vi "KPropertyTable Test.vi"() -> ()   [LabVIEW 2020]
uses:
  KPropertyTable/RowData.ctl
  KPropertyTable/DataType.ctl
  KPropertyTable/KPropertyTable.xctl
panel:
  out "data":T1
  in  "stop":bool
  in  "Table":T2[](xcontrol)
  out "Rows":T2[](array[typedef])
  in  "props":T1
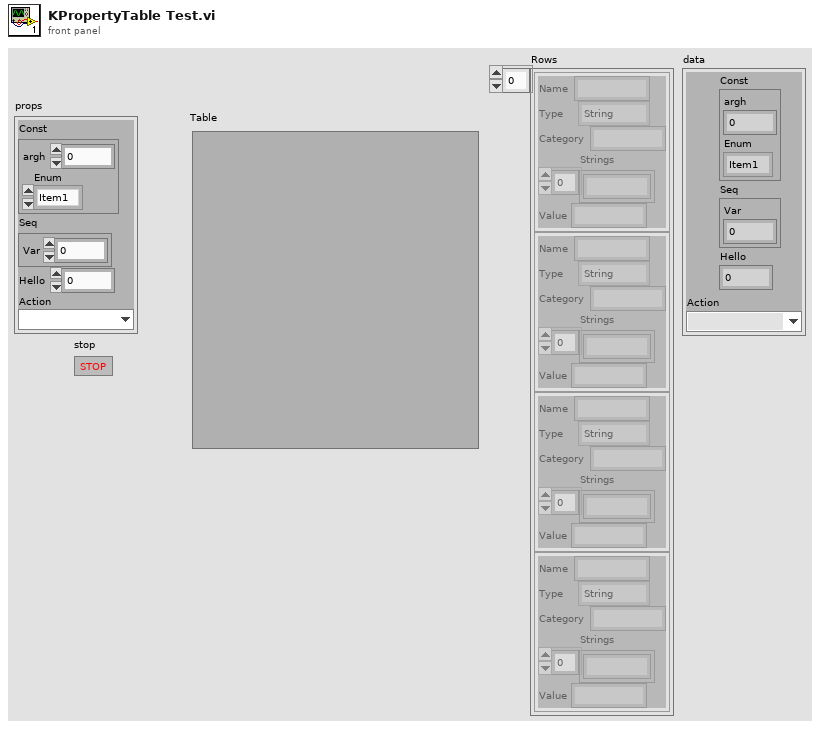
[diagram p1: front panel]
types:
  T1 = cluster{"Const":cluster{"argh":dbl, "Enum":enum16{"Item1", "ItermB"}}, "Seq":cluster{"Var":dbl}, "Hello":i32, "Action":enum16{""}}
  T2 = typedef "KPropertyTable.xctl/RowData.ctl" = cluster{"Name":string, "Type":T3, "Category":string, "Strings":string[], "Value":string}
  T3 = typedef "KPropertyTable.xctl/DataType.ctl" = enum16{"String", "Enum", "Int", "Double", "Boolean", "Ring", "Formula"}
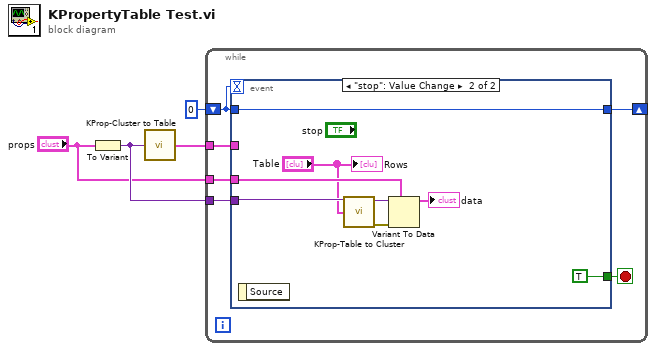
[diagram p0: block diagram]
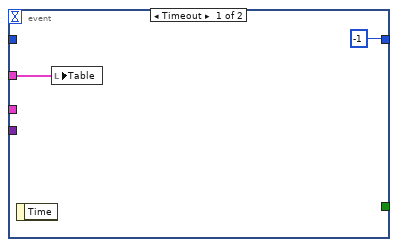
[diagram p2: hidden frame]
diagram:
  n1 = To Variant(anything="props") -> (Variant=w2:variant)
  n2 = call "KProp-Cluster to Table.vi"("Anything"=w2) -> ("Rows"=w4:T2[])  [unwired: 13 in, 1 out]
  n3 = while {
    tunnel: w4 -> [w10]
    shift-right: [w8] -> _
    shift-left: 0 -> [w9]
    tunnel: w2 -> [w6]
    tunnel: "props" -> [w5]
    stop <- w7 stop-if-true
    n4 = event shown="[1] \"stop\": Value Change" {
      selector: _ -> [_ _]
      dyn-events: _ -> [_ _]
      timeout: w9 -> [_ _]
      tunnel: w10 -> [w12 _]
      tunnel: w9 -> [_ w20]
      tunnel: [-1 w20] -> w8
      tunnel: [_ TRUE] -> w7
      tunnel: w6 -> [_ w17]
      tunnel: w5 -> [_ w18]
      event Timeout {
        n5 = event-data() -> ()  [unwired: 1 in, 1 out]
        n6 = local write "Table"(w12) -> ()
      }
      event "stop": Value Change {
        n7 = event-data() -> ()  [unwired: 1 in, 1 out]
        n8 = call "KProp-Table to Cluster.vi"("Anything"=w17, "Rows"="Table") -> ("variant"=w14:variant, "Error Out"=w15:errorcluster)  [unwired: 12 in]
        n9 = Variant To Data(error in=w15, type=w18, Variant=w14) -> (data=→"data":T1)  [unwired: 1 out]
        "Rows" <- "Table"
      }
    }
  }
